vi "Initialize TCS Stream.vi"(8 "error in (no error)":errorcluster, 10 "TCS Simulated/Real":bool, 11 "TCS in":refnum<class "TCS.lvclass">) -> (0 "error out":errorcluster, 3 "TCS out":refnum<class "TCS.lvclass">)   [LabVIEW 2018, in "TCS.lvclass"]
uses:
  TCS.lvclass
  TCS.lvclass/TCS.ctl
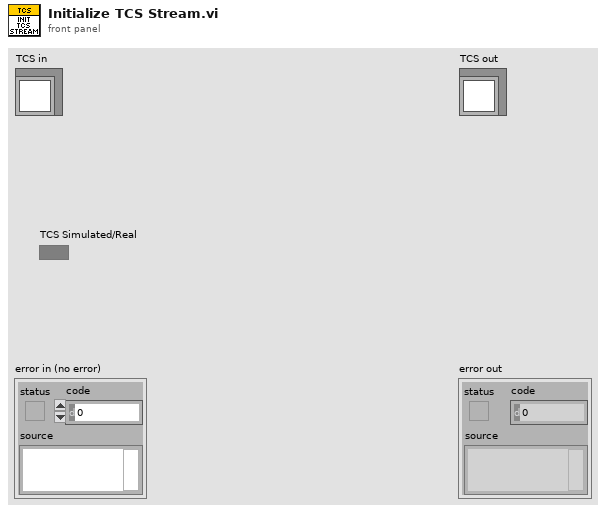
[diagram p1: front panel]
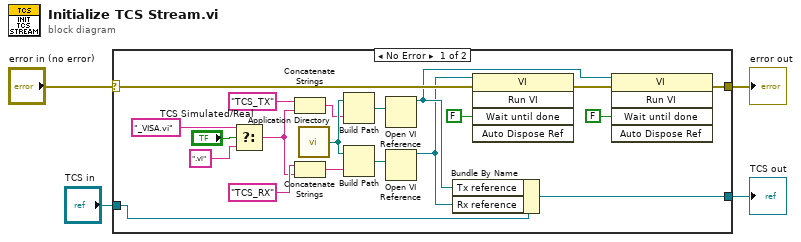
[diagram p0: block diagram]
diagram:
  n1 = case shown="No Error" "error in (no error)" {
    selector: "error in (no error)" -> [w18 w26]
    tunnel: [w17 w26] -> w3
    tunnel: [w15 w25] -> w1
    tunnel: "TCS in" -> [w16 w25]
    frame No Error {
      n2 = Select(t="_VISA.vi", s="TCS Simulated/Real", f=".vi") -> (s? t:f=w9:string)
      n3 = Concatenate Strings("TCS_TX", w9) -> (w7:string)
      n4 = Concatenate Strings("TCS_RX", w9) -> (w8:string)
      n5 = call <vilib>:"Application Directory.vi"() -> ("Application Directory"=w20:path)
      n6 = Build Path(base path=w20, name or relative path=w7) -> (appended path=w21:path)
      n7 = Build Path(base path=w20, name or relative path=w8) -> (appended path=w24:path)
      n8 = Open VI Reference(vi path=w21) -> (vi reference=w14:refnum<vi>)  [unwired: 5 in, 1 out]
      n9 = Open VI Reference(vi path=w24) -> (vi reference=w13:refnum<vi>)  [unwired: 5 in, 1 out]
      n10 = Bundle By Name(cluster=w16, "Tx reference"=w14, "Rx reference"=w13) -> (w15:refnum<class "TCS.lvclass">)
      n11 = invoke class="VI" method="Run VI"(reference=w13, error in=w18, "Wait until done"=FALSE ("Wait Until Done")) -> (error out=w19:errorcluster)  [unwired: 2 in, 4 out]
      n12 = invoke class="VI" method="Run VI"(reference=w14, error in=w19, "Wait until done"=FALSE ("Wait Until Done")) -> (error out=w17:errorcluster)  [unwired: 2 in, 4 out]
    }
    frame Error {
    }
  }
  "error out" <- w3
  "TCS out" <- w1
